vi "nanocal frontend client 19.vi"() -> ()   [LabVIEW 2019]
uses:
  frontend -- data type.ctl
panel:
  in  "shared variable refnum in":refnum<k21>
  out "data out":T1
  in  "stop":bool
  in  "milliseconds to wait":u32=100
  out "Numeric":i32
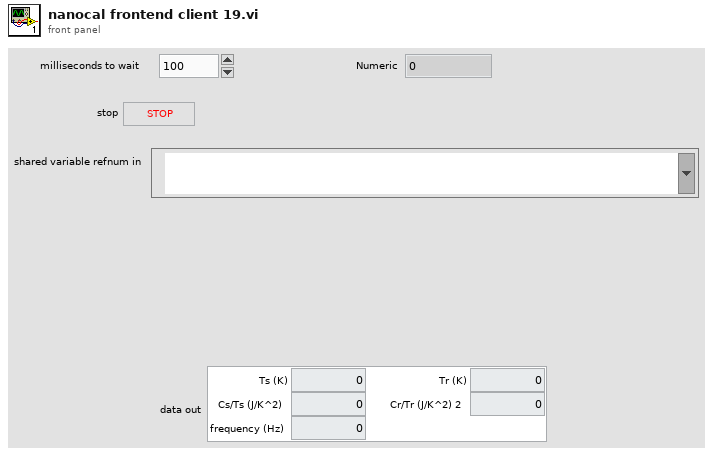
[diagram p1: front panel]
types:
  T1 = typedef "frontend -- data type.ctl" = cluster{"frequency (Hz)":dbl, "Cs/Ts (J/K^2)":dbl, "Ts (K)":dbl, "Cr/Tr (J/K^2) 2":dbl, "Tr (K)":dbl}
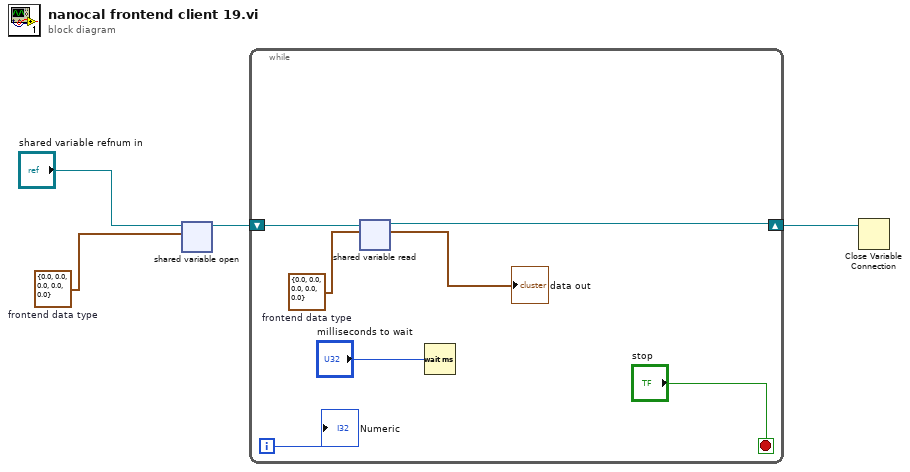
[diagram p0: block diagram]
diagram:
  w2 = T1 {"frequency (Hz)"=0.0, "Cs/Ts (J/K^2)"=0.0, "Ts (K)"=0.0, "Cr/Tr (J/K^2) 2"=0.0, "Tr (K)"=0.0}  # frontend data type
  n1 = shared-variable-open("shared variable refnum in", w2) -> (w4:refnum<k21>)  [unwired: 2 in, 1 out]
  n2 = while {
    shift-right: [w5] -> w3
    shift-left: w4 -> [w8]
    i -> [w11]
    stop <- "stop" stop-if-true
    w7 = T1 {"frequency (Hz)"=0.0, "Cs/Ts (J/K^2)"=0.0, "Ts (K)"=0.0, "Cr/Tr (J/K^2) 2"=0.0, "Tr (K)"=0.0}  # frontend data type
    n3 = shared-variable-read(w8, w7) -> (w5:refnum<k21>, →"data out":T1)  [unwired: 1 in, 2 out]
    n4 = Wait (ms)(milliseconds to wait="milliseconds to wait") -> ()  [unwired: 1 out]
    "Numeric" <- w11
  }
  n5 = Close Variable Connection(11:w3) -> ()  [unwired: 1 in, 1 out]
